vi "求方程的根（两分法）.vi"() -> ()   [LabVIEW 2012]
doc: "功能：\n\n利用牛顿迭代法求一个数的n次方根\n\n\ncsxcs_366创建"
panel:
  in  "区间b-":dbl
  out "根":dbl
  in  "区间a+":dbl
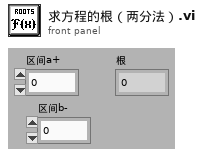
[diagram p1: front panel]
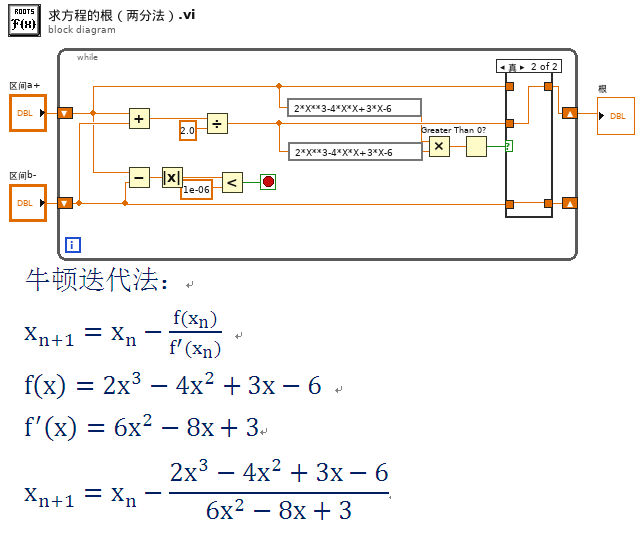
[diagram p0: block diagram]
diagram:
  n1 = while {
    shift-right: [w11] -> w1
    shift-left: "区间a+" -> [w4]
    shift-right: [w12] -> _
    shift-left: "区间b-" -> [w5]
    stop <- w16 stop-if-true
    n2 = Add(x=w4, y=w5) -> (x+y=w15:dbl)
    n3 = Subtract(x=w4, y=w5) -> (x-y=w6:dbl)
    n4 = Absolute Value(x=w6) -> (abs(x)=w18:dbl)
    n5 = Divide(x=w15, y=2.0) -> (x/y=w10:dbl)
    n6 = Less?(x=w18, y=1e-06) -> (x < y?=w16:bool)
    n7 = expression code="2*X**3-4*X*X+3*X-6"(w4) -> (w9:dbl)
    n8 = expression code="2*X**3-4*X*X+3*X-6"(w10) -> (w8:dbl)
    n9 = Multiply(x=w9, y=w8) -> (x*y=w7:dbl)
    n10 = Greater Than 0?(x=w7) -> (x > 0?=w13:bool)
    n11 = case shown="真" w13 {
      tunnel: w4 -> [w20 _]
      tunnel: w5 -> [_ w22]
      tunnel: w10 -> [w19 w21]
      tunnel: [w19 w22] -> w12
      tunnel: [w20 w21] -> w11
      frame False {
      }
      frame True {
      }
    }
  }
  "根" <- w1
